vi "Get Element and Attributes from Tag.vi"(8 "error in (no error)":errorcluster, 11 "tag with attributes":string) -> (0 "error out":errorcluster, 2 "Attributes":cluster{"Keys":string[], "Values":string[]}, 3 "element name":string, 5 "empty element?":bool)   [LabVIEW 2011]
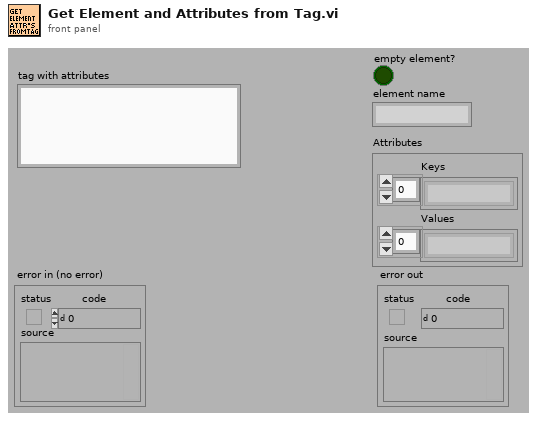
[diagram p1: front panel]
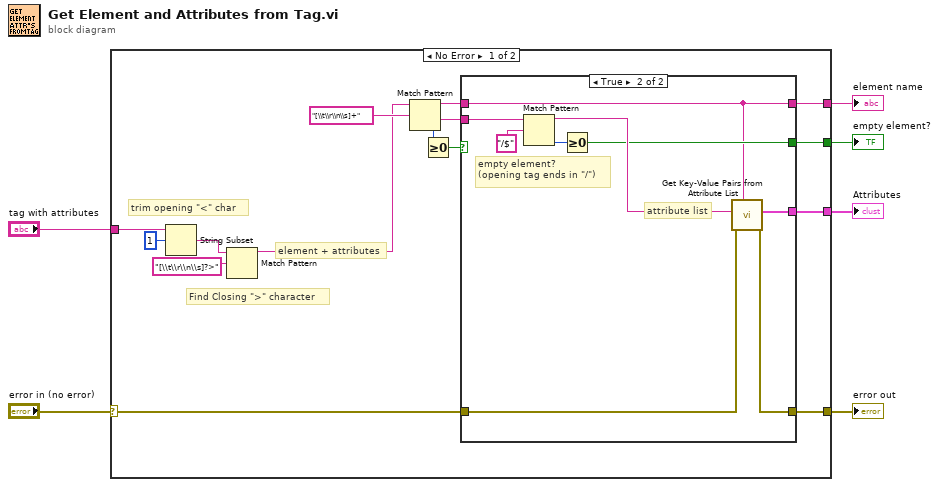
[diagram p0: block diagram]
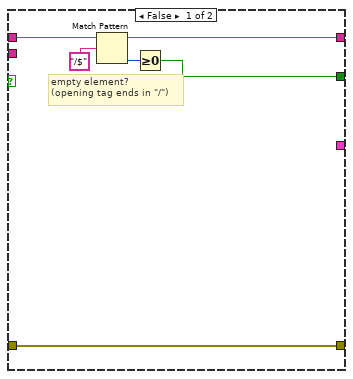
[diagram p2: hidden frame]
diagram:
  n1 = case shown="No Error" "error in (no error)" {
    selector: "error in (no error)" -> [w8 w37]
    tunnel: "tag with attributes" -> [w17 _]
    tunnel: [w9 _] -> w5
    tunnel: [w13 _] -> w1
    tunnel: [w14 _] -> w4
    tunnel: [w7 w37] -> w2
    frame No Error {
      # "element + attributes"
      # "Find Closing \">\" character"
      # "trim opening \"<\" char"
      n2 = String Subset(string=w17, offset (0)=1) -> (substring=w19:string)  [unwired: 1 in]
      n3 = Match Pattern(string=w19, regular expression="[\\t\\r\\n\\s]?>") -> (before substring=w16:string)  [unwired: 1 in, 3 out]
      n4 = Match Pattern(string=w16, regular expression="[\\t\\r\\n\\s]+") -> (before substring=w10:string, after substring=w15:string, offset past match=w12:i32)  [unwired: 1 in, 1 out]
      n5 = Greater Or Equal To 0?(x=w12) -> (x >= 0?=w11:bool)
      n6 = case shown="True" w11 {
        tunnel: w15 -> [_ w35]
        tunnel: [w25 w32] -> w14
        tunnel: [_ w31] -> w13
        tunnel: [w23 w28] -> w9
        tunnel: w10 -> [w24 w28]
        tunnel: w8 -> [w22 w30]
        tunnel: [w22 w29] -> w7
        frame False {
          # "empty element?\n(opening tag ends in \"/\")"
          n7 = Match Pattern(string=w24, regular expression="/$") -> (before substring=w23:string, offset past match=w26:i32)  [unwired: 1 in, 2 out]
          n8 = Greater Or Equal To 0?(x=w26) -> (x >= 0?=w25:bool)
        }
        frame True {
          # "attribute list"
          # "empty element?\n(opening tag ends in \"/\")"
          n9 = Match Pattern(string=w35, regular expression="/$") -> (before substring=w34:string, offset past match=w33:i32)  [unwired: 1 in, 2 out]
          n10 = Greater Or Equal To 0?(x=w33) -> (x >= 0?=w32:bool)
          n11 = call "Get Key-Value Pairs from Attribute List.vi"("element name (for errors)"=w28, "error in (no error)"=w30, "attribute list"=w34) -> ("error out"=w29:errorcluster, "attributes"=w31:cluster{"name":string[], "value":string[]})  [unwired: 7 in]
        }
      }
    }
    frame Error {
    }
  }
  "element name" <- w5
  "Attributes" <- w1
  "empty element?" <- w4
  "error out" <- w2
